vi "Write Probe Attenuation.vi"(8 "error in (no error)":errorcluster, 10 "Probe Attenuation":dbl, 11 "Osciloscope in":refnum<class "Osciloscope.lvclass">) -> (0 "error out":errorcluster, 3 "Osciloscope out":refnum<class "Osciloscope.lvclass">)   [LabVIEW 2020, in "Osciloscope Tektronix.lvlib" / "Osciloscope.lvclass"]
uses:
  Osciloscope.lvclass
  Osciloscope.lvclass/Osciloscope.ctl
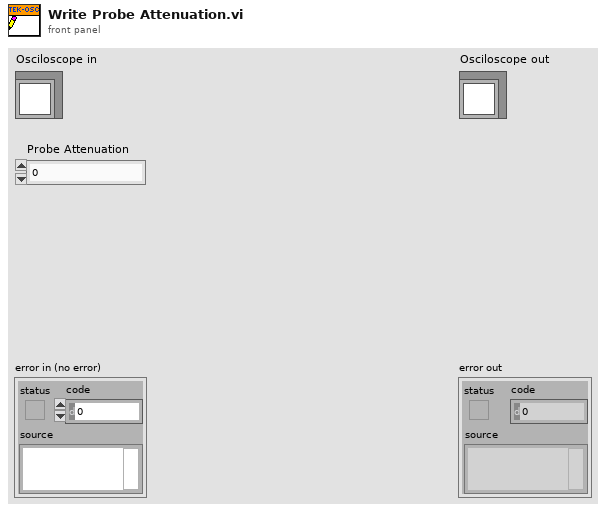
[diagram p1: front panel]
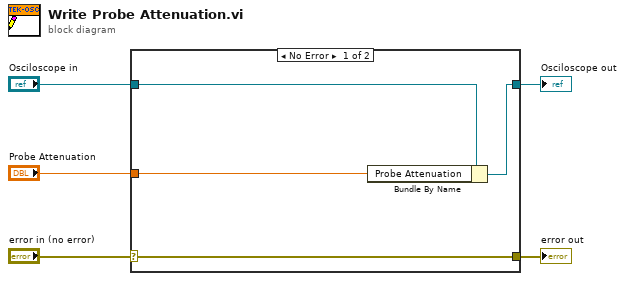
[diagram p0: block diagram]
diagram:
  n1 = case shown="No Error" "error in (no error)" {
    selector: "error in (no error)" -> [w9 w10]
    tunnel: [w9 w10] -> w4
    tunnel: [w7 w11] -> w2
    tunnel: "Osciloscope in" -> [w8 w11]
    tunnel: "Probe Attenuation" -> [w6 _]
    frame No Error {
      n2 = Bundle By Name(cluster=w8, "Probe Attenuation"=w6) -> (w7:refnum<class "Osciloscope.lvclass">)
    }
    frame Error {
    }
  }
  "error out" <- w4
  "Osciloscope out" <- w2
